vi "Init Sync Stuff.vi"(8 "error in (no error)":errorcluster, 10 "Template in":refnum<class "Template.lvclass">) -> (0 "error out":errorcluster, 2 "Template out":refnum<class "Template.lvclass">)   [LabVIEW 2011, in "Tinkerforge.lvlib" / "Template.lvclass"]
doc: "This VI is the child implementation of \"Init Sync Stuff.vi\" and initializes all synchronization objects of this child object."
uses:
  Template.lvclass
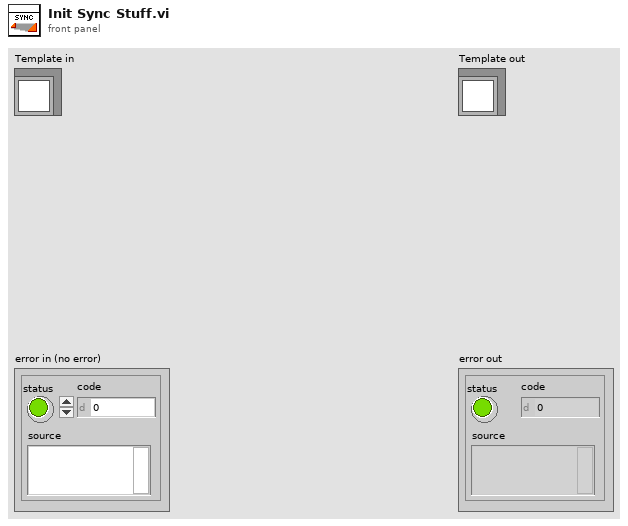
[diagram p1: front panel]
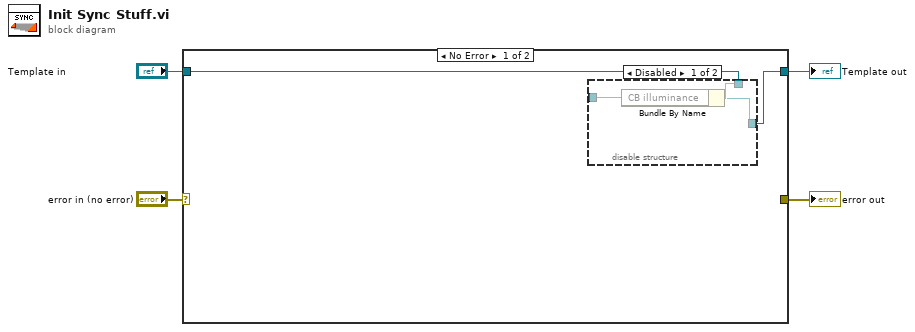
[diagram p0: block diagram]
diagram:
  n1 = case shown="No Error" "error in (no error)" {
    selector: "error in (no error)" -> [_ w11]
    tunnel: "Template in" -> [w6 w12]
    tunnel: [_ w11] -> w2
    tunnel: [w5 w12] -> w1
    frame No Error {
      n2 = disable-structure shown="Disabled" {
        disable-tunnel: w6 -> [w9 w10]
        disable-tunnel: [w8 w10] -> w5
        disable-tunnel: _ -> [w7 _]
        frame Disabled {
          n3 = Bundle By Name(cluster=w9, "CB illuminance"=w7) -> (w8:refnum<class "Template.lvclass">)
        }
        frame Enabled {
        }
      }
    }
    frame Error {
    }
  }
  "error out" <- w2
  "Template out" <- w1
